vi "getClassHierarchy.vi"(8 "error in":errorcluster, 10 "className":string) -> (0 "error out":errorcluster, 2 "classHierarchy":string[](array[string]))   [LabVIEW 2020, in "JKI JSON Object Serialization.lvlib" / "OOP_Utility.lvlib" / "Reflection.lvclass"]
doc: "Get the class hierarchy for the specified class. The first element of the output array is the top most parent class; the last element is the input class. Input className can include or exclude the '.lvclass' extension. Output values include '.lvclass' extension.\n\nGCraftsman JSON Object Serialization Toolkit\nwww.GCraftsman.com\nCopyright (c) 2017, GCraftsman"
uses:
  Reflection.lvclass
  reflectionPoolAction.ctl
  Reflection.lvclass/Reflection.ctl
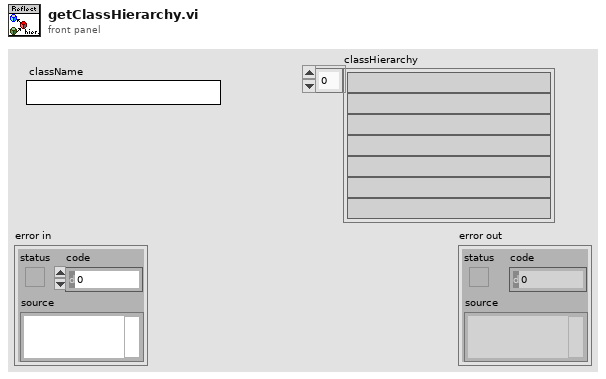
[diagram p1: front panel]
types:
  T1 = typedef "JKI JSON Object Serialization.lvlib/OOP_Utility.lvlib/Reflection.lvclass/reflectionPoolAction.ctl" = enum16{"<select>", "getPrivateData", "getClassHierarchy", "getClassVersions", "getAllClasses"}
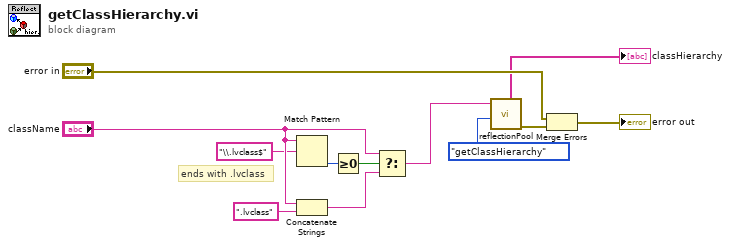
[diagram p0: block diagram]
diagram:
  # "ends with .lvclass"
  n1 = Match Pattern(string="className", regular expression="\\.lvclass$") -> (offset past match=w10:i32)  [unwired: 1 in, 3 out]
  n2 = Concatenate Strings("className", ".lvclass" ("regular expression")) -> (w6:string)
  n3 = Greater Or Equal To 0?(x=w10) -> (x >= 0?=w9:bool)
  n4 = Select(t="className", s=w9, f=w6) -> (s? t:f=w1:string)
  n5 = call "reflectionPool.vi"("action"=reflectionPoolAction."getClassHierarchy", "class name"=w1) -> ("error out"=w5:errorcluster, "class hierarchy"=→"classHierarchy":string[])  [unwired: 4 in, 4 out]
  n6 = Merge Errors("error in", w5) -> (→"error out":errorcluster)
